vi "Initialise.vi"(8 "error in (no error)":errorcluster, 10 "Buses":refnum<class "Bus_Access.lvclass">[](array[class]), 11 "Fault-Injection Bus in":refnum<class "Fault-Injection Bus.lvclass">) -> (0 "error out":errorcluster, 3 "Fault-Injection Bus out":refnum<class "Fault-Injection Bus.lvclass">)   [LabVIEW 2021, in "Fault-Injection Bus.lvclass"]
uses:
  Fault-Injection Bus.lvclass
  Omni-Bus/Bus Access/Bus_Access.lvclass
  Fault-Injection Bus.lvclass/Fault-Injection Bus.ctl
  Properties/Write Buses.vi
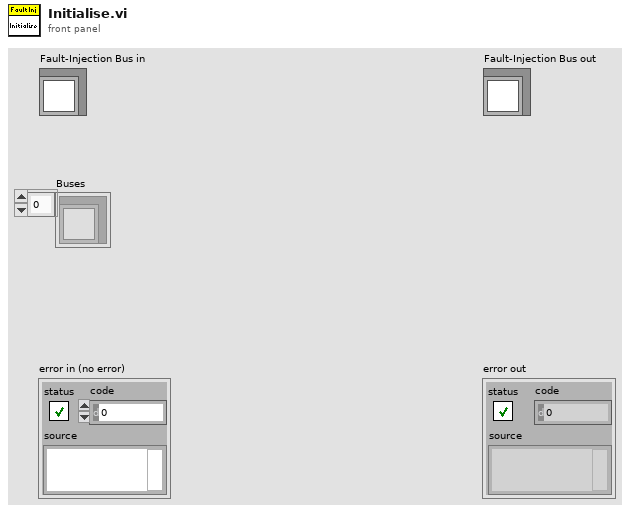
[diagram p1: front panel]
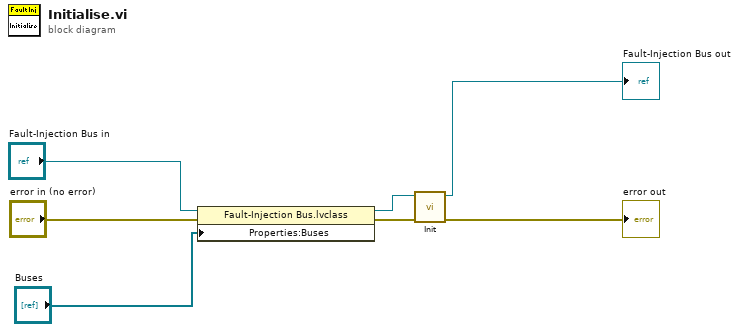
[diagram p0: block diagram]
diagram:
  n1 = property class="Fault-Injection Bus.lvclass"(reference="Fault-Injection Bus in", error in="error in (no error)", "Properties:Buses"="Buses") -> (reference out=w3:refnum<class "Fault-Injection Bus.lvclass">, error out=w4:errorcluster)
  n2 = call-dynamic "Init.vi"("error in (no error)"=w4, "Data in"=w3) -> ("error out"=→"error out":errorcluster, "Data out"=→"Fault-Injection Bus out":refnum<class "Fault-Injection Bus.lvclass">)  [unwired: 8 in]
